vi "AI Start.vi"(8 "error in (no error)":errorcluster, 11 "NI Analog Input in":refnum<class "NI Analog Input.lvclass">) -> (0 "error out":errorcluster, 3 "NI Analog Input out":refnum<class "NI Analog Input.lvclass">)   [LabVIEW 2020, in "NI DAQmx.lvlib" / "NI Analog Input.lvclass"]
uses:
  NI Analog Input.lvclass
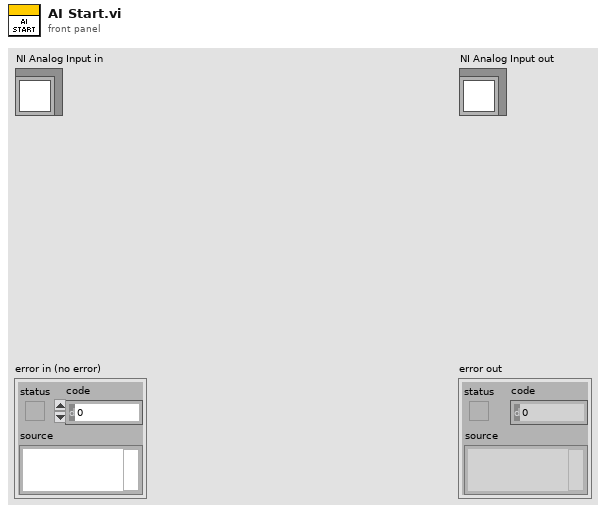
[diagram p1: front panel]
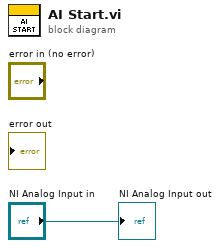
[diagram p0: block diagram]
diagram:
  "NI Analog Input out" <- "NI Analog Input in"
